vi "HP 3437A III.vi"(4 "trigger mode":i16(slide) scale=0.0..2.0, 5 "range (10V:2)":i16(slide)=2 scale=0.0..2.0 scale format="%.2f") -> (0 "AVE":dbl=1.9939)   [LabVIEW 2010]
doc: "HP 3437A DC Voltmeter\n\nUse: measure dc volts on three different ranges.\n\nDefaults: 10.0V range (input = 2), Internal trigger (input = 0), 0 second Delay, N = 1.\n\nOptions not included: the ability to set and use hold/manual triggering.\n\nAssumptions: the GPIB address is 24, the bus is properly connected.\n\n\nTo use this Virtual Instrument interactively, set the range as desired, choose the desired triggering mode, set the delay (0 to 0.9999999 seconds), and choose the number of readings (1 to 9999) to be returned in the output array (labeled 'Output'). If only one reading is desired, set N to 1 and obtain the output from the scalar output (labeled 'Output(0)'). This output is the first element in the array, and thus it is the only element when N is set to 1.\n\nTo use this Virtual Instrument programmatically, set the delay time to a desired default (or rewire the connector pane). Then provide inputs for the Range, Trigger Mode, and N controls. The inputs for the Range and Trigger Mode controls are as shown:\n\n Range: 0 = 0.1V Trigger Mode: 0 = Internal\n 1 = 1.0V 1 = External; imd.\n 2 = 10.0V 2 = External; wait\n\nThe outputs are as above--use the scalar output if only one reading is desired, use the array output if multiple readings are desired.\n\nWhen an array output is desired, several different parameters need to be considered. The most important parameter is the timeout value for the interface boards. To insure that there is enough time to return all the data, the product of N and Delay, N*Delay, is computed. If the value is less than 60, the timeout is set to 60 seconds. If, however, the product is greater than 60, the timeout is set to that value, provided that the product is less than 3600, which is the maximum. If N*Delay is greater than 3600 seconds, a warning is issued and execution of the VI halts. If this situation arises, adjust N and/or Delay accordingly. The other parameter to be considered is the triggering mode desired. If external triggering is desired, there are two options provided by the VI. The first option (\"External; imd.\") starts the read immediately after the voltmeter is set up. This mode should be used if it is mandatory that the first readings be returned, but it will only return M values, where M is such that M*Delay ² 60 seconds. The other option (\"External; wait\") waits until the trigger has been received to begin the read. This mode should be used if N*Delay > 60 seconds. However, be warned that if the delay time is smaller than about 0.05 to 0.06 seconds, a considerable amount of data will be lost. (This driver is designed to give maximum throughput by the voltmeter, thus causing data to be overwritten--and lost--unless the read is started immediately after the set up.) In the range of 0.05 to 0.06 seconds, 1-10 readings may be lost, while any delay time greater than 0.06 seconds should return every reading. If N*Delay > 60 seconds and it is necessary to obtain the first values measured but delay time cannot be increased, the \"low end\" timeout value can be increased, provided this value does not exceed 3600 seconds.\n\nInstrument overflow, which is indicated by ±0.9999, ±9.999, or ±99.99 on the voltmeter, is indicated by ±0.1999, ±1.999, or ±19.99, respectively on the Virtual Instrument. Data is valid in all other cases (except as noted above), i.e., 1.998 is a valid reading when the range is set to 1.0V.\n\nNote: InitVI must be run with Xon/Xoff set to off (false) and buffer size set to at least 2*N.\n \n\nThis VI sets the HP 3437A voltmeter up to read N readings using a specified delay. The first reading in the output array is returned as a scalar in case only one value is needed.\nversion a.0"
panel:
  out "Waveform Chart":ext(graph)=1.9939000000000000004
  out "counts":dbl=3.0
  in  "# points":dbl=100.0
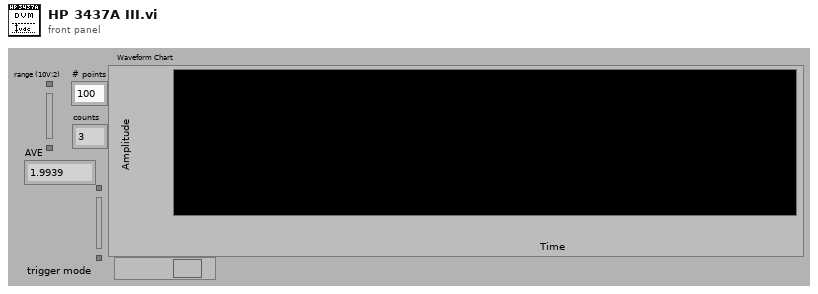
[diagram p1: front panel]
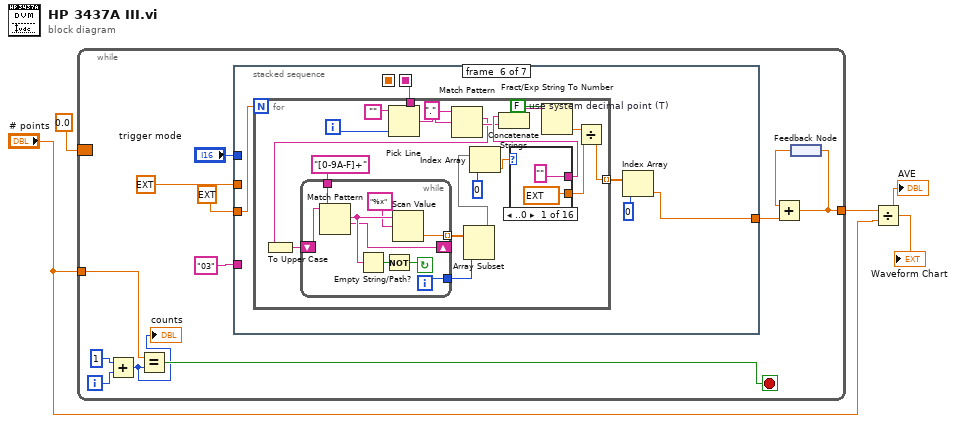
[diagram p0: block diagram]
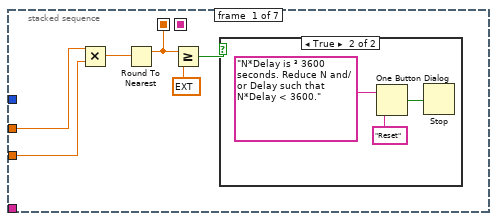
[diagram p2: hidden frame]
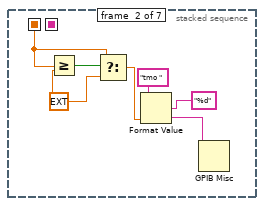
[diagram p4: hidden frame]
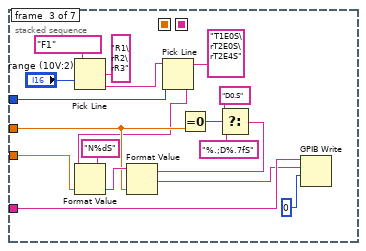
[diagram p5: hidden frame]
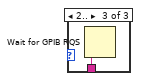
[diagram p8: hidden frame]
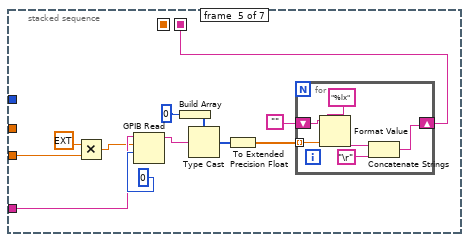
[diagram p9: hidden frame]
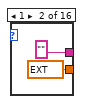
[diagram p10: hidden frame]
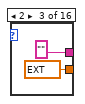
[diagram p11: hidden frame]
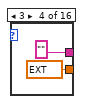
[diagram p12: hidden frame]
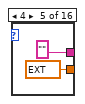
[diagram p13: hidden frame]
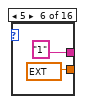
[diagram p14: hidden frame]
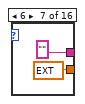
[diagram p15: hidden frame]
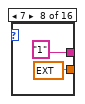
[diagram p16: hidden frame]
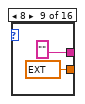
[diagram p17: hidden frame]
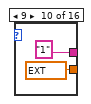
[diagram p18: hidden frame]
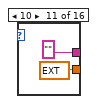
[diagram p19: hidden frame]
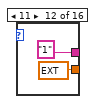
[diagram p20: hidden frame]
diagram:
  n1 = while {
    tunnel: "# points" -> [w10]
    tunnel: [w6] -> w3
    border: 0.0 -> [_]
    i -> [w11]
    stop <- w9 stop-if-true
    n2 = Add(x=1, y=w11) -> (x+y=w5:i32)
    "counts" <- w5
    n3 = Equal?(x=w10, y=w5) -> (x = y?=w9:bool)
    n4 = stacked-sequence {
      seq-local: [w21 _ _ _ _ _ _] -> [_ w28 _ _ _ _ _]
      seq-local: [_ _ _ _ w58 _ _] -> [_ _ _ _ _ w73 _]
      tunnel: "03" -> [_ _ w34 w52 w56 _ _]
      tunnel: ext 1.0 ("N") -> [w19 _ w38 _ w65 w76 _]
      tunnel: ext 0.0 ("delay") -> [w20 _ w48 _ _ _ _]
      tunnel: "trigger mode" -> [_ _ w39 w51 _ _ _]
      tunnel: [_ _ _ _ _ w72 _] -> w8
      frame #0 {
        n5 = Multiply(x=w20, y=w19) -> (x*y=w18:ext)
        n6 = Round To Nearest(number=w18) -> (nearest integer value=w21:ext)
        n7 = Greater Or Equal?(x=w21, y=ext 3600.0) -> (x >= y?=w17:bool)
        n8 = case shown="True" w17 {
          frame False {
          }
          frame True {
            n9 = One Button Dialog(message="N*Delay is ³ 3600 seconds. Reduce N and/or Delay such that N*Delay < 3600.", button name ("OK")="Reset") -> (true=w23:bool)
            n10 = Stop(stop? (T)=w23) -> ()
          }
        }
      }
      frame #1 {
        w29 = ext 60.0
        n11 = Greater Or Equal?(x=w28, y=w29) -> (x >= y?=w30:bool)
        n12 = Select(t=w28, s=w30, f=w29) -> (s? t:f=w31:ext)
        n13 = Format Value(string ("")="tmo ", format string="%d", value (0)=w31) -> (output string=w27:string)
        n14 = GPIB Misc(0:w27) -> ()  [unwired: 1 in, 3 out]
      }
      frame #2 {
        n15 = Pick Line(string ("")="F1", multi-line string="R1\rR2\rR3", line index="range (10V:2)") -> (output string=w40:string)
        n16 = Pick Line(string ("")=w40, multi-line string="T1E0S\rT2E0S\rT2E4S", line index=w39) -> (output string=w36:string)
        n17 = Format Value(string ("")=w36, format string="N%dS", value (0)=w38) -> (output string=w49:string)
        n18 = Equal To 0?(x=w48) -> (x = 0?=w45:bool)
        n19 = Select(t="D0.S", s=w45, f="%.;D%.7fS") -> (s? t:f=w50:string)
        n20 = Format Value(string ("")=w49, format string=w50, value (0)=w48) -> (output string=w33:string)
        n21 = GPIB Write(0:w34, 1:w33, 2:0) -> ()  [unwired: 1 in, 3 out]
      }
      frame #3 {
        n22 = case shown="..0" w51 {
          tunnel: w52 -> [_ _ w53]
          frame ..0 {
          }
          frame 1 {
          }
          frame 2.. {
            n23 = Wait for GPIB RQS(4:w53) -> ()  [unwired: 1 in, 3 out]
          }
        }
      }
      frame #4 {
        n24 = Multiply(x=ext 2.0, y=w65) -> (x*y=w55:ext)
        n25 = GPIB Read(0:w56, 1:w55, 2:0) -> (5:w54:string)  [unwired: 1 in, 3 out]
        n26 = Build Array(u16 0) -> (w63:u16[])
        n27 = Type Cast(type=w63, x=w54) -> (*(type *) &x=w62:u16[])
        n28 = To Extended Precision Float(1:w62) -> (0:w59:ext[])
        n29 = for {
          shift-right: [w69] -> w58
          shift-left: "" -> [w70]
          tunnel: w59 -> [w68] mode=indexing
          n30 = Format Value(string ("")=w70, format string="%lx", value (0)=w68) -> (output string=w71:string)
          n31 = Concatenate Strings(w71, "\r") -> (w69:string)
        }
      }
      frame #5 {
        n32 = for {
          N: w76 -> [_]
          tunnel: w73 -> [w82]
          tunnel: [w96] -> w74 mode=indexing
          i -> [w89]
          (unwired) FALSE ("use system decimal point (T)")
          w77 = FALSE  # use system decimal point (T)
          n33 = Pick Line(string ("")="", multi-line string=w82, line index=w89) -> (output string=w91:string)
          n34 = Match Pattern(string=w91, regular expression=".") -> (match substring=w79:string, after substring=w92:string)  [unwired: 3 out]
          n35 = To Upper Case(1:w79) -> (0:w81:string)
          n36 = while {
            tunnel: [w103] -> w84
            tunnel: [w102] -> w83 mode=indexing
            tunnel: "[0-9A-F]+" -> [w98]
            shift-left: w81 -> [w101]
            shift-right: [w99] -> _
            i -> [w103]
            stop <- w105 continue-if-true
            n37 = Match Pattern(string=w101, regular expression=w98) -> (match substring=w100:string, after substring=w99:string)  [unwired: 3 out]
            n38 = Empty String/Path? ("Empty String?")(string/path=w100) -> (empty?=w104:bool)
            n39 = Not(x=w104) -> (.not. x?=w105:bool)
            n40 = Scan Value(string=w100, format string="%x") -> (value=w102:dbl)  [unwired: 2 out]
          }
          n41 = Array Subset(array=w83, length=w84) -> (w80:dbl[])  [unwired: 1 in]
          n42 = Index Array(array=w80, index=0) -> (element=w86:dbl)
          n43 = case shown="..0" w86 {
            tunnel: ["" "" "" "" "" "1" "" "1" "" "1" "" "1" "" "1" "" "1"] -> w93
            tunnel: [ext 1e+99 ext 1e+99 ext 1e+99 ext 1e+99 ext -10000.0 ext -10000.0 ext 10000.0 ext 10000.0 ext -100.0 ext -1e+21 ext 100.0 ext 100.0 ext -1000.0 ext -1000.0 ext 1000.0 ext 1000.0] -> w95
            frame ..0 {
            }
            frame 1 {
            }
            frame 2 {
            }
            frame 3 {
            }
            frame 4 {
            }
            frame 5 {
            }
            frame 6 {
            }
            frame 7 {
            }
            frame 8 {
            }
            frame 9 {
            }
            frame 10 {
            }
            frame 11 {
            }
            frame 12 {
            }
            frame 13 {
            }
            frame 14 {
            }
            frame 15.. {
            }
          }
          n44 = Concatenate Strings(w93, w92) -> (w94:string)
          n45 = Fract/Exp String To Number(use system decimal point (T)=w77, string=w94) -> (number=w85:dbl)  [unwired: 3 out]
          n46 = Divide(x=w85, y=w95) -> (x/y=w96:ext)
        }
        n47 = Index Array(array=w74, index=0) -> (element=w72:ext)
      }
      frame #6 {
        n48 = GPIB Misc(0:"tmo 10") -> ()  [unwired: 1 in, 3 out]
      }
    }
    n49 = feedback #1() -> (w7:ext)
    n50 = Add(x=w7, y=w8) -> (x+y=w6:ext)
    n51 = feedback-in #1(w6) -> ()
  }
  n52 = Divide(x=w3, y="# points") -> (x/y=→"AVE" →"Waveform Chart":ext)
